vi "IT8800-Configure Response Speed.vi"(8 "error in":errorcluster, 10 "Response Speed":u16(ring) items=["Normal Response Speed", "1/2 the Normal Response Speed", "1/5 the Normal Response Speed", "1/10 the Normal Response Speed"], 11 "IT8800 Setting In In":T1={"VISA Resource Name"="", "Baud Rate"=19200, "Stop Bits"=20, "Wait For Read(ms)"=0, "Interface Type"=enum."GPIB", "Limits"=[]} {"Stop Bits" items=["1.0"=10, "2.0"=20]; "Baud Rate" items=["2400"=2400, "4800"=4800, "9600"=9600, "19200"=19200]}) -> (0 "error out":errorcluster, 3 "IT8800 Setting In Out":T1={"VISA Resource Name"="", "Baud Rate"=19200, "Stop Bits"=20, "Wait For Read(ms)"=0, "Interface Type"=enum."GPIB", "Limits"=[]} {"Stop Bits" items=["1.0"=10, "2.0"=20]; "Baud Rate" items=["2400"=2400, "4800"=4800, "9600"=9600, "19200"=19200]})   [LabVIEW 2018]
doc: "Configures the response speed of the instrument. The PLZ4W operates by detecting the input current or voltage and feeding back those values. You can decrease the response speed to assure stable operation.\n\n<b>Note:</b>\n1) Works in CC,CR, CC+CV and CR+CV mode."
uses:
  Data Def/IT8800-Setting.ctl
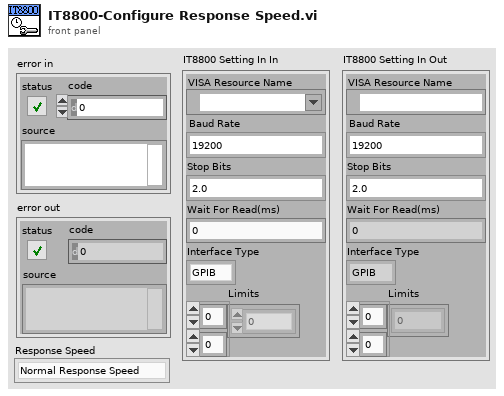
[diagram p1: front panel]
types:
  T1 = typedef "IT8800-Setting.ctl" = cluster{"VISA Resource Name":refnum<visa-resource-name>, "Baud Rate":u32, "Stop Bits":u16, "Wait For Read(ms)":u32, "Interface Type":enum16{"Unknow", "GPIB", "VXI", "GPIB-VXI", "Serial", "PXI", "TCPIP", "USB", "FireWire"}, "Limits":dbl[][]}
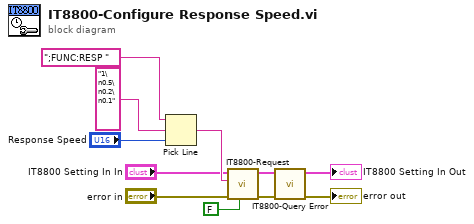
[diagram p0: block diagram]
diagram:
  n1 = Pick Line(string ("")=";FUNC:RESP ", multi-line string="1\n0.5\n0.2\n0.1", line index="Response Speed") -> (output string=w4:string)
  n2 = call "IT8800-Request.vi"("Response?"=FALSE, "error in"="error in", "Command"=w4, "IT8800 Setting In In"="IT8800 Setting In In") -> ("error out"=w7:errorcluster, "IT8800 Setting In Out"=w6:T1)  [unwired: 5 in, 1 out]
  n3 = call "IT8800-Query Error.vi"("error in"=w7, "IT8800 Setting In In"=w6) -> ("error out"=→"error out":errorcluster, "IT8800 Setting In Out"=→"IT8800 Setting In Out":T1)  [unwired: 8 in]
